vi "SetProcessDefault.vi"(8 "error in (no error)":errorcluster, 11 "Logger in":refnum<class "Logger.lvclass">) -> (0 "error out":errorcluster)   [LabVIEW 2026, in "Lumberjack.lvlib"]
uses:
  Lumberjack.lvlib
  Public/Logger.lvclass/Logger.lvclass
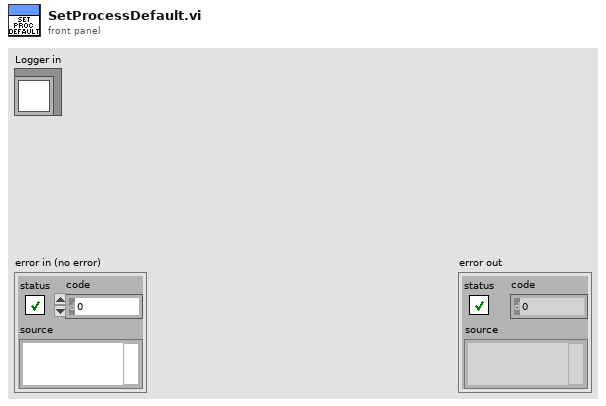
[diagram p1: front panel]
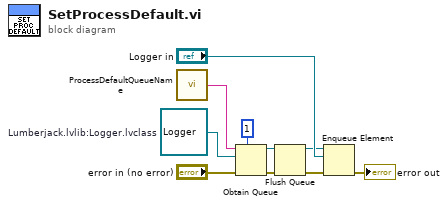
[diagram p0: block diagram]
diagram:
  w3 = refnum<class "Logger.lvclass"> refnum  # Lumberjack.lvlib:Logger.lvclass
  n1 = call "ProcessDefaultQueueName.vi"() -> ("processDefaultQueueName"=w6:string)
  n2 = Obtain Queue(max queue size (-1, unlimited)=1, name (unnamed)=w6, element data type=w3, error in (no error)="error in (no error)") -> (queue out=w7:refnum<queue>, error out=w9:errorcluster)  [unwired: 1 in, 1 out]
  n3 = Flush Queue(queue=w7, error in (no error)=w9) -> (queue out=w1:refnum<queue>, error out=w5:errorcluster)  [unwired: 1 out]
  n4 = Enqueue Element(queue=w1, element="Logger in", error in (no error)=w5) -> (error out=→"error out":errorcluster)  [unwired: 1 in, 2 out]
